vi "Initialize Default FPGA Bitfile.vi"(8 "error in (no error)":errorcluster) -> (0 "error out":errorcluster)   [LabVIEW 2021, in "Utilities.lvlib"]
uses:
  <vilib>/myRIO/Instrument Drivers/Utilities/Utilities.lvlib
  <vilib>/userdefined/High Color/nirio_resource_hc.ctl
panel:
  # "Opens a reference to the myRIO hardware"
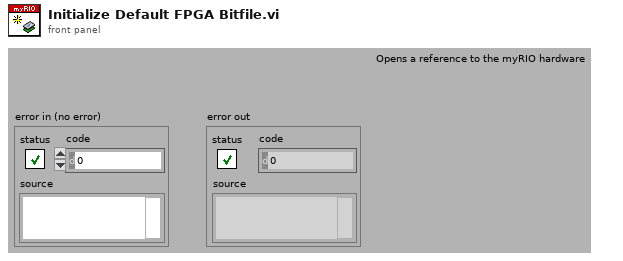
[diagram p1: front panel]
types:
  T1 = typedef "nirio_resource_hc.ctl" = tag
  T2 = typedef "Hardware Version Enum.ctl" = enum16{"Unknown", "myRIO-1900", "myRIO-1950", "roboRIO", "NI ELVIS RIO CM", "ELVIS III"}
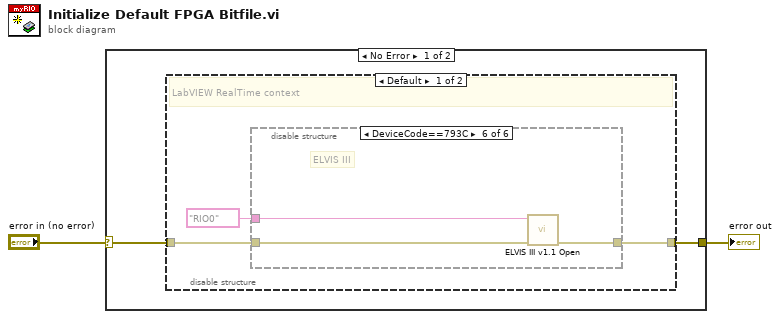
[diagram p0: block diagram]
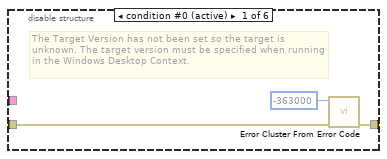
[diagram p2: hidden frame]
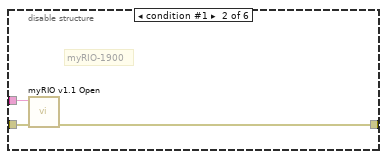
[diagram p3: hidden frame]
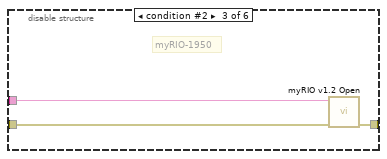
[diagram p4: hidden frame]
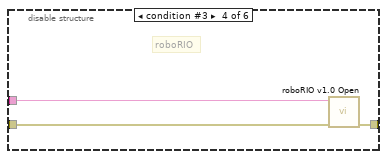
[diagram p5: hidden frame]
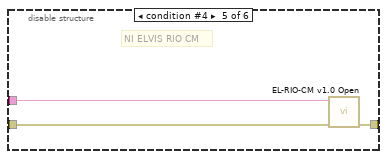
[diagram p6: hidden frame]
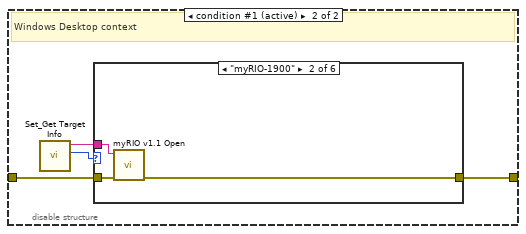
[diagram p7: hidden frame]
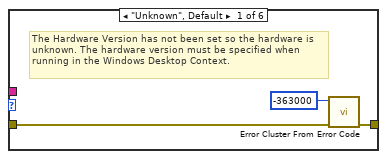
[diagram p8: hidden frame]
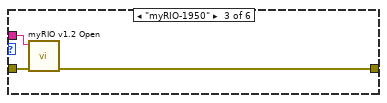
[diagram p9: hidden frame]
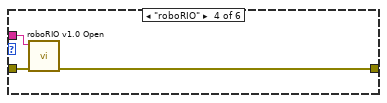
[diagram p10: hidden frame]
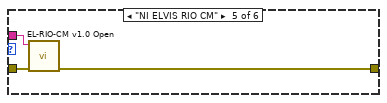
[diagram p11: hidden frame]
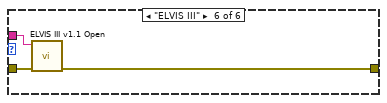
[diagram p12: hidden frame]
diagram:
  n1 = case shown="No Error" "error in (no error)" {
    selector: "error in (no error)" -> [w3 w48]
    tunnel: [w4 w48] -> w2
    frame No Error {
      n2 = disable-structure shown="Default" {
        disable-tunnel: [w7 w29] -> w4
        disable-tunnel: w3 -> [w6 w28]
        frame condition #0 {
          # "LabVIEW RealTime context"
          n3 = disable-structure shown="DeviceCode==793C" {
            disable-tunnel: [w10 w11 w14 w17 w20 w25] -> w7
            disable-tunnel: w6 -> [w9 w12 w15 w18 w21 w23]
            disable-tunnel: T1 "RIO0" ("Resource name") -> [_ w13 w16 w19 w22 w24]
            frame condition #0 (active) {
              # "The Target Version has not been set so the target is unknown. The target version must be specified when running in the Windows Desktop Context."
              n4 = call <vilib>:"Error Cluster From Error Code.vi"("error in (no error)"=w9, "error code (0)"=-363000) -> ("error out"=w10:errorcluster)  [unwired: 7 in]
            }
            frame condition #1 {
              # "myRIO-1900"
              n5 = call <vilib>:"myRIO v1.1 Open.vi"("error in (no error)"=w12, "Resource name"=w13) -> ("error out"=w11:errorcluster)  [unwired: 8 in, 1 out]
            }
            frame condition #2 {
              # "myRIO-1950"
              n6 = call <vilib>:"myRIO v1.2 Open.vi"("error in (no error)"=w15, "Resource name"=w16) -> ("error out"=w14:errorcluster)  [unwired: 8 in, 1 out]
            }
            frame condition #3 {
              # "roboRIO"
              n7 = call <vilib>:"roboRIO v1.0 Open.vi"("error in (no error)"=w18, "Resource name"=w19) -> ("error out"=w17:errorcluster)  [unwired: 8 in, 1 out]
            }
            frame condition #4 {
              # "NI ELVIS RIO CM"
              n8 = call <vilib>:"EL-RIO-CM v1.0 Open.vi"("error in (no error)"=w21, "Resource name"=w22) -> ("error out"=w20:errorcluster)  [unwired: 8 in, 1 out]
            }
            frame condition #5 {
              # "ELVIS III"
              n9 = call <vilib>:"ELVIS III v1.1 Open.vi"("error in (no error)"=w23, "Resource name"=w24) -> ("error out"=w25:errorcluster)  [unwired: 8 in, 1 out]
            }
          }
        }
        frame condition #1 (active) {
          # "Windows Desktop context"
          n10 = call <vilib>:"Set_Get Target Info.vi"() -> ("Hardware Version"=w26:T2, "IP Address"=w27:string)  [unwired: 9 in, 1 out]
          n11 = case shown="\"myRIO-1900\"" w26 {
            tunnel: [w32 w33 w36 w39 w42 w46] -> w29
            tunnel: w28 -> [w30 w34 w38 w41 w44 w47]
            tunnel: w27 -> [_ w35 w37 w40 w43 w45]
            frame "Unknown", Default {
              # "The Hardware Version has not been set so the hardware is unknown. The hardware version must be specified when running in the Windows Desktop Context."
              n12 = call <vilib>:"Error Cluster From Error Code.vi"("error in (no error)"=w30, "error code (0)"=-363000) -> ("error out"=w32:errorcluster)  [unwired: 7 in]
            }
            frame "myRIO-1900" {
              n13 = call <vilib>:"myRIO v1.1 Open.vi"("error in (no error)"=w34, "Resource name"=w35) -> ("error out"=w33:errorcluster)  [unwired: 8 in, 1 out]
            }
            frame "myRIO-1950" {
              n14 = call <vilib>:"myRIO v1.2 Open.vi"("error in (no error)"=w38, "Resource name"=w37) -> ("error out"=w36:errorcluster)  [unwired: 8 in, 1 out]
            }
            frame "roboRIO" {
              n15 = call <vilib>:"roboRIO v1.0 Open.vi"("error in (no error)"=w41, "Resource name"=w40) -> ("error out"=w39:errorcluster)  [unwired: 8 in, 1 out]
            }
            frame "NI ELVIS RIO CM" {
              n16 = call <vilib>:"EL-RIO-CM v1.0 Open.vi"("error in (no error)"=w44, "Resource name"=w43) -> ("error out"=w42:errorcluster)  [unwired: 8 in, 1 out]
            }
            frame "ELVIS III" {
              n17 = call <vilib>:"ELVIS III v1.1 Open.vi"("error in (no error)"=w47, "Resource name"=w45) -> ("error out"=w46:errorcluster)  [unwired: 8 in, 1 out]
            }
          }
        }
      }
    }
    frame Error {
    }
  }
  "error out" <- w2
